vi "DoWrite.vi"(8 "error in (no error)":errorcluster, 9 "Value":u32 format="%.0x", 10 "Register Address":u32 format="%.0x", 11 "VISA Reference":refnum<visa-resource-name>) -> (0 "error out":errorcluster, 3 "dup VISA resource name":refnum<visa-resource-name>)   [LabVIEW 2016]
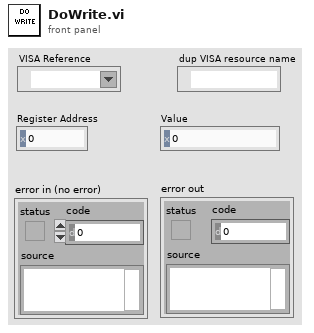
[diagram p1: front panel]
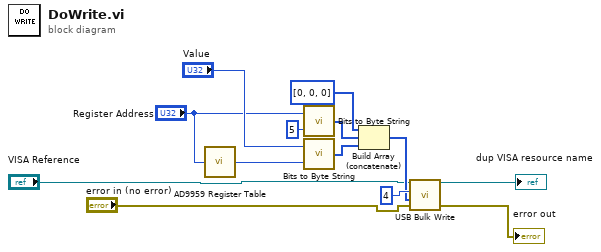
[diagram p0: block diagram]
diagram:
  n1 = call "AD9959 Register Table.vi"("Register Address"="Register Address") -> ("Register Width"=w10:i32)
  n2 = call "Bits to Byte String.vi"("width"=5, "Value"="Register Address") -> ("Byte String"=w8:u8[])
  n3 = call "Bits to Byte String.vi"("width"=w10, "Value"="Value") -> ("Byte String"=w7:u8[])
  n4 = Build Array (concatenate)(u8[] [0, 0, 0], w8, w7) -> (w5:u8[])
  n5 = call "USB Bulk Write.vi"("error in (no error)"="error in (no error)", "message"=w5, "Endpoint"=i16 4, "VISA Reference"="VISA Reference") -> ("error out"=→"error out":errorcluster, "dup VISA resource name"=→"dup VISA resource name":refnum<visa-resource-name>)  [unwired: 1 out]
